vi "二阶重建数据准备.vi"(0 "关联成像原理":dbl, 1 "少量采样数据M":i32, 5 "重建方法":dbl, 7 "优化算法":dbl, 9 "光源散斑簇":T1, 11 "图像簇":T2) -> (4 "照射差分求和数组":dbl[](array[numeric]), 6 "正图像筛选门限":dbl)   [LabVIEW 2018]
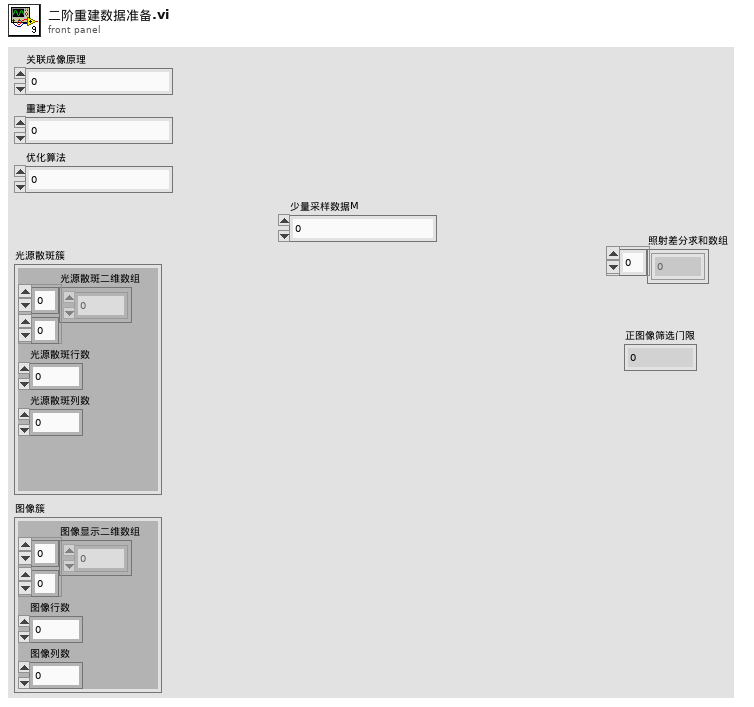
[diagram p1: front panel]
types:
  T1 = cluster{"光源散斑二维数组":dbl[][], "光源散斑行数":i32, "光源散斑列数":i32}
  T2 = cluster{"图像显示二维数组":dbl[][], "图像行数":i32, "图像列数":i32}
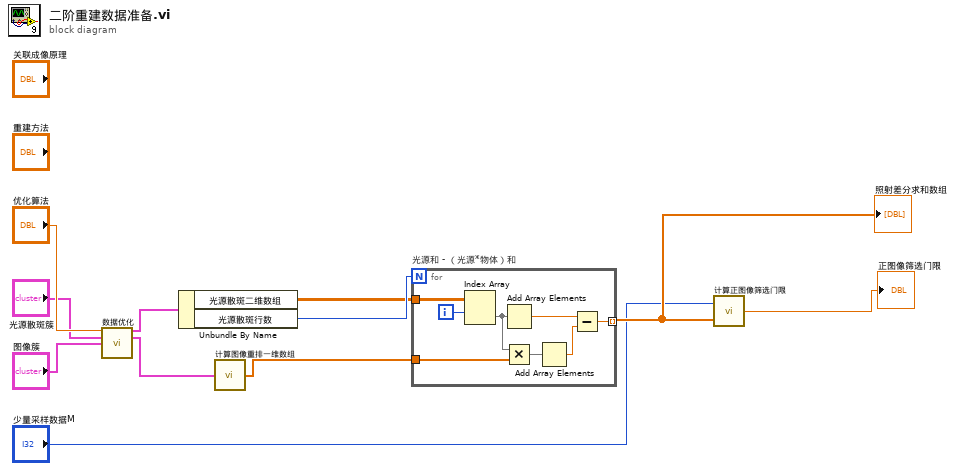
[diagram p0: block diagram]
diagram:
  n1 = call "数据优化.vi"("优化算法"="优化算法", "光源散斑簇"="光源散斑簇", "图像簇"="图像簇") -> ("优化光源散斑簇"=w3:T1, "优化图像簇"=w1:T2)  [unwired: 11 in]
  n2 = Unbundle By Name(w3) -> ("光源散斑二维数组"=w9:dbl[][], "光源散斑行数"=w11:i32)
  n3 = call "计算图像重排一维数组.vi"("优化图像簇"=w1) -> ("图像重排一维数组"=w10:dbl[])
  n4 = for "光源和 - （光源*物体）和" {
    N: w11 -> [_]
    tunnel: w9 -> [w19]
    tunnel: w10 -> [w18]
    tunnel: [w14] -> w8 mode=indexing
    i -> [w13]
    n5 = Index Array(array=w19, index (row)=w13) -> (element=w16:dbl[])  [unwired: 1 in]
    n6 = Add Array Elements(numeric array=w16) -> (sum=w12:dbl)
    n7 = Multiply(x=w16, y=w18) -> (x*y=w17:dbl[])
    n8 = Add Array Elements(numeric array=w17) -> (sum=w15:dbl)
    n9 = Subtract(x=w12, y=w15) -> (x-y=w14:dbl)
  }
  "照射差分求和数组" <- w8
  n10 = call "计算正图像筛选门限.vi"("差分计算一维矩阵"=w8, "少量采样数据量"="少量采样数据M") -> ("正图像筛选门限"=→"正图像筛选门限":dbl)
